vi "Write FPLocation.vi"(3 "(FPPos)":refnum<class "Frame_FPPos.lvclass">, 4 "FPLocation":T1) -> (5 "(FPPos) Out":refnum<class "Frame_FPPos.lvclass">)   [LabVIEW 2016, in "Frame_FPPos.lvclass"]
uses:
  Frame_FPPos.lvclass
  TypeDefs_Utility/ENUM RB_Pos_Quadrant Position.ctl
  Frame_FPPos.lvclass/Frame_FPPos.ctl
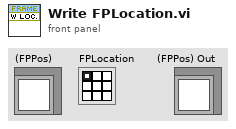
[diagram p1: front panel]
types:
  T1 = typedef "ENUM RB_Pos_Quadrant Position.ctl" = enum32{"LFT-TOP", "MID-TOP", "RGT-TOP", "LFT-CTR", "MID-CTR", "RGT-CTR", "LFT-BOT", "MID-BOT", "RGT-BOT"}
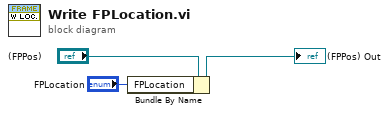
[diagram p0: block diagram]
diagram:
  n1 = Bundle By Name(cluster="(FPPos)", "FPLocation"="FPLocation") -> (→"(FPPos) Out":refnum<class "Frame_FPPos.lvclass">)
